vi "Load Tiff image from data.vi"(8 "Litt/BigEnd":bool, 9 "DirEntries":T1[](array[typedef]), 11 "Image Data in":u8[](array[numeric])) -> (1 "N_Bits":u64, 2 "Gray16/32":sgl[][](array[numeric]))   [LabVIEW 2013, in "Tiff reader.lvlib"]
doc: "This .vi loads a Tiff image from file."
uses:
  Tiff reader.lvlib
  IFD Entry.ctl
  FieldTypes.ctl
panel:
  in  "Tab Control":T3(tab)
  out "Gray8":u8[][](array[numeric])
  out "Grayscale":picture
  out "Gray8 LUT":u8[][](array[numeric])
  out "GrayWithLUT":picture
  out "RGB8":u32[][](array[numeric])
  out "B16/32":sgl[][](array[numeric])
  out "G16/32":sgl[][](array[numeric])
  out "R16/32":sgl[][](array[numeric])
  out "N_RGB_Bits":u64
  out "RGB":picture
  in  "error in (no error)":errorcluster
  out "error out":errorcluster
  out "PhotoM":T4(ring)=enum."BlackIsZero"
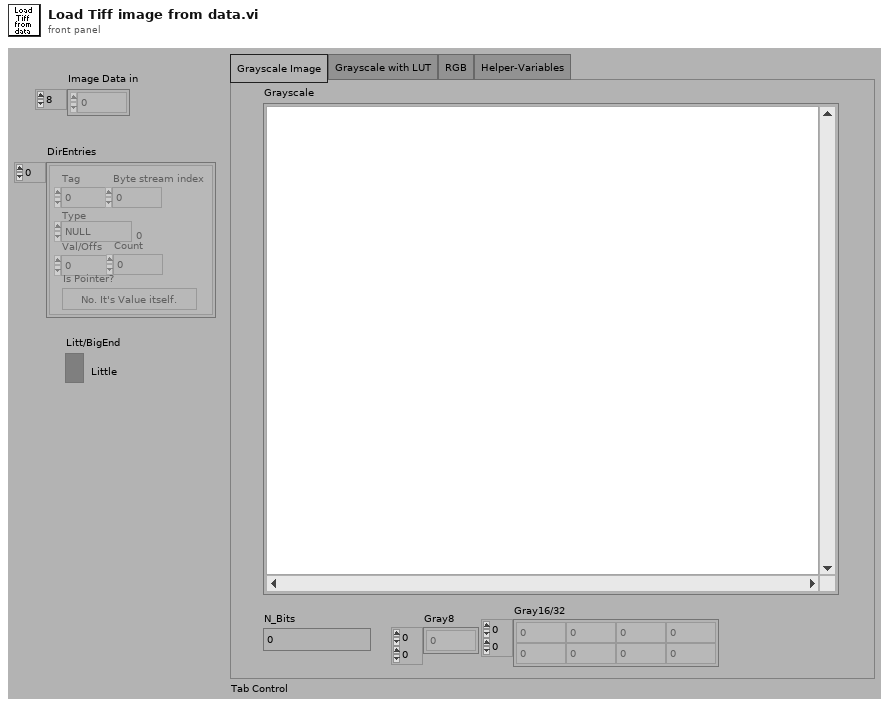
[diagram p1: front panel]
types:
  T1 = typedef "Tiff reader.lvlib/IFD Entry.ctl" = cluster{"Tag":u16, "Type":T2, "Count":u32, "Val/Offs":u32, "Is Pointer?":bool, "Byte stream index":i32}
  T2 = typedef "Tiff reader.lvlib/FieldTypes.ctl" = enum16{"NULL", "U8", "ASCII7", "U16", "U32", "RATIONAL", "SByte(I8)", "Undef(8Bit)", "I16", "I32", "SRat(4B:4B)", "SGL(4Byte)", "DBL(8Byte)"}
  T3 = enum32{"Grayscale Image", "Grayscale with LUT", "RGB", "Helper-Variables"}
  T4 = enum16{"WhiteIsZero", "BlackIsZero", "RGB", "RGBPalette", "TranspMask", "CMYK", "YCbCr", "Null", "CIELab"}
  T5 = typedef "imagedata.ctl" = cluster{"image type":i32, "image depth":i32, "image":u8[], "mask":u8[], "colors":u32[], "Rectangle":cluster{"left":i16, "top":i16, "right":i16, "bottom":i16}}
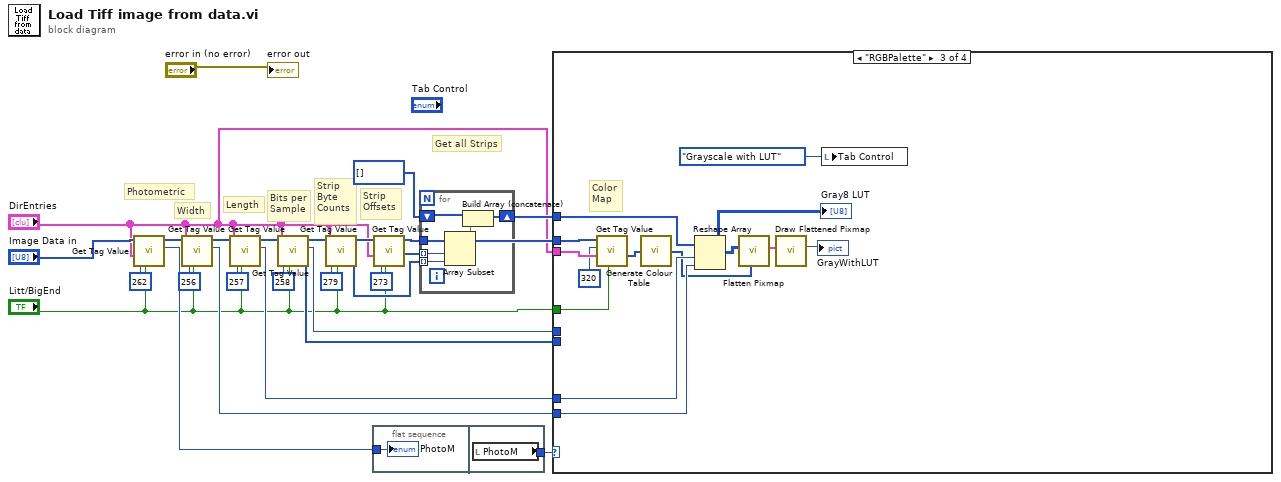
[diagram p0: block diagram]
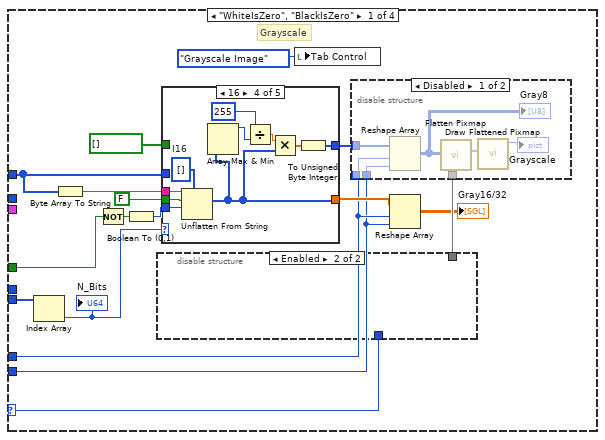
[diagram p2: hidden frame]
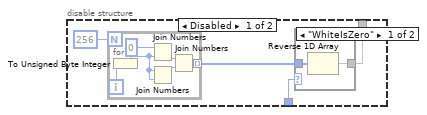
[diagram p3: hidden frame]
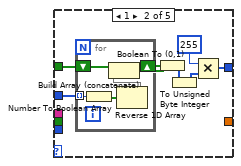
[diagram p7: hidden frame]
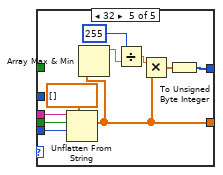
[diagram p9: hidden frame]
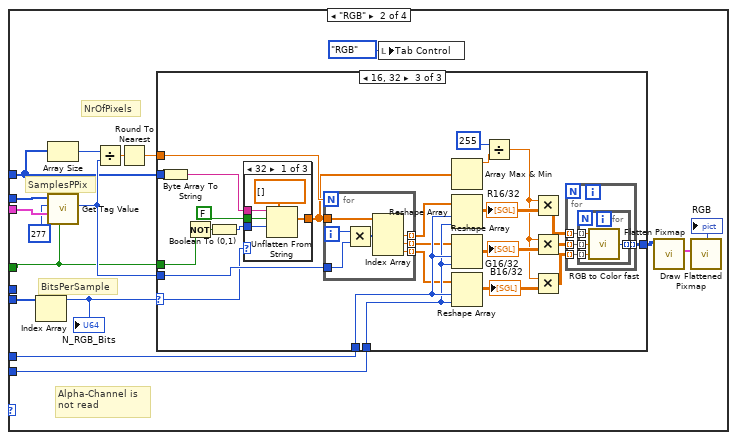
[diagram p10: hidden frame]
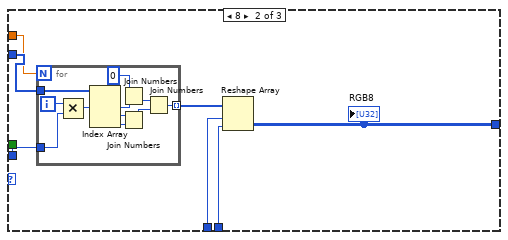
[diagram p12: hidden frame]
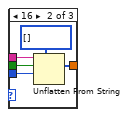
[diagram p13: hidden frame]
diagram:
  # "Get all Strips"
  # "Strip\nOffsets"
  # "Strip\nByte\nCounts"
  # "Bits per\nSample"
  # "Photometric"
  # "Length"
  # "Width"
  n1 = call "Get Tag Value.vi"("Litt/BigEnd"="Litt/BigEnd", "DirEntries"="DirEntries", "Tag Code"=u16 262, "Image Data in"="Image Data in") -> ("Single Value"=w11:u32, "Image Data out"=w21:u8[])  [unwired: 4 out]
  n2 = call "Get Tag Value.vi"("Litt/BigEnd"="Litt/BigEnd", "DirEntries"="DirEntries", "Tag Code"=u16 256, "Image Data in"=w21) -> ("Single Value"=w22:u32, "Image Data out"=w26:u8[])  [unwired: 4 out]
  n3 = call "Get Tag Value.vi"("Litt/BigEnd"="Litt/BigEnd", "DirEntries"="DirEntries", "Tag Code"=u16 257, "Image Data in"=w26) -> ("Single Value"=w23:u32, "Image Data out"=w18:u8[])  [unwired: 4 out]
  n4 = call "Get Tag Value.vi"("Litt/BigEnd"="Litt/BigEnd", "DirEntries"="DirEntries", "Tag Code"=u16 258, "Image Data in"=w18) -> ("Multiple Values"=w12:u64[], "Single Value"=w13:u32, "Image Data out"=w17:u8[])  [unwired: 3 out]
  n5 = call "Get Tag Value.vi"("Litt/BigEnd"="Litt/BigEnd", "DirEntries"="DirEntries", "Tag Code"=u16 279, "Image Data in"=w17) -> ("Multiple Values"=w7:u64[], "Image Data out"=w16:u8[])  [unwired: 4 out]
  n6 = flat-sequence {
    tunnel: w11 -> [w27]
    tunnel: [w28] -> w10
    frame #0 {
      "PhotoM" <- w27
    }
    frame #1 {
      n7 = local read "PhotoM"() -> (w28:T4)
    }
  }
  n8 = call "Get Tag Value.vi"("Litt/BigEnd"="Litt/BigEnd", "DirEntries"="DirEntries", "Tag Code"=u16 273, "Image Data in"=w16) -> ("Multiple Values"=w8:u64[], "Image Data out"=w9:u8[])  [unwired: 4 out]
  n9 = for {
    tunnel: w9 -> [w34]
    tunnel: w8 -> [w33] mode=indexing
    tunnel: w7 -> [w32] mode=indexing
    shift-right: [w31] -> w5
    shift-left: u8[] [] -> [w29]
    n10 = Array Subset(array=w34, index=w33, length=w32) -> (w30:u8[])
    n11 = Build Array (concatenate)(w29, w30) -> (w31:u8[])
  }
  n12 = case shown="\"RGBPalette\"" w10 {
    selector: w10 -> [w42 _ _ _]
    tunnel: w23 -> [w41 w121 w197 _]
    tunnel: w9 -> [_ w119 w199 _]
    tunnel: w22 -> [w40 w120 w196 _]
    tunnel: "DirEntries" -> [_ w118 w202 _]
    tunnel: w13 -> [_ _ _ _]
    tunnel: w12 -> [w47 w116 _ _]
    tunnel: w5 -> [w46 w107 w195 _]
    tunnel: "Litt/BigEnd" -> [w37 w105 w190 _]
    frame "WhiteIsZero", "BlackIsZero" {
      # "Grayscale"
      n13 = Index Array(array=w47) -> (element=w39:u64)  [unwired: 1 in]
      "N_Bits" <- w39
      n14 = Byte Array To String(unsigned byte array=w46) -> (string=w51:string)
      n15 = Not(x=w37) -> (.not. x?=w48:bool)
      n16 = Boolean To (0,1)(Boolean=w48) -> (0, 1=w49:i16)
      n17 = disable-structure shown="Enabled" {
        disable-tunnel: [w53 _] -> w43
        disable-tunnel: w42 -> [w52 _]
        frame Disabled {
          n18 = for {
            N: 256 -> [_]
            tunnel: [w59] -> w54 mode=indexing
            i -> [w64]
            n19 = To Unsigned Byte Integer(number=w64) -> (unsigned 8bit integer=w62:u8)
            n20 = Join Numbers(hi=u8 0, lo=w62) -> ((hi.lo)=w60:u16)
            n21 = Join Numbers(hi=w62, lo=w62) -> ((hi.lo)=w61:u16)
            n22 = Join Numbers(hi=w60, lo=w61) -> ((hi.lo)=w59:u32)
          }
          n23 = case shown="\"WhiteIsZero\"" w52 {
            tunnel: w54 -> [w57 w58]
            tunnel: [w56 w58] -> w53
            frame "WhiteIsZero" {
              n24 = Reverse 1D Array(array=w57) -> (reversed array=w56:u32[])
            }
            frame "BlackIsZero", Default {
            }
          }
        }
        frame Enabled {
        }
      }
      n25 = case shown="16" w39 {
        tunnel: w51 -> [_ _ _ w94 w103]
        tunnel: [_ _ w84 w85 w96] -> w44
        tunnel: FALSE ("data includes array or string size? (T)") -> [_ _ _ w93 w102]
        tunnel: w49 -> [_ _ _ w92 w101]
        tunnel: w46 -> [_ w78 w84 _ _]
        tunnel: [_ w73 w84 w86 w97] -> w45
        tunnel: bool[] [] -> [_ w72 _ _ _]
        frame 0, 4, Default {
          # "not\nsupported"
        }
        frame 1 {
          n26 = for {
            tunnel: w78 -> [w83] mode=indexing
            shift-right: [w82] -> w77
            shift-left: w72 -> [w81]
            n27 = Number To Boolean Array(number=w83) -> (Boolean array=w80:bool[])
            n28 = Reverse 1D Array(array=w80) -> (reversed array=w79:bool[])
            n29 = Build Array (concatenate)(w81, w79) -> (w82:bool[])
          }
          n30 = Boolean To (0,1)(Boolean=w77) -> (0, 1=w76:i16[])
          n31 = To Unsigned Byte Integer(number=w76) -> (unsigned 8bit integer=w75:u8[])
          n32 = Multiply(x=u8 255, y=w75) -> (x*y=w73:u8[])
        }
        frame 8 {
        }
        frame 16 {
          w91 = i16[] []  # I16
          n33 = Unflatten From String(type=w91, binary string=w94, data includes array or string size? (T)=w93, byte order (0:big-endian, network order)=w92) -> (value=w85:i16[])  [unwired: 1 in, 2 out]
          n34 = Array Max & Min(array=w85) -> (max value=w90:i16)  [unwired: 3 out]
          n35 = Divide(x=255 ("Numeric"), y=w90) -> (x/y=w89:dbl)
          n36 = Multiply(x=w89, y=w85) -> (x*y=w87:dbl[])
          n37 = To Unsigned Byte Integer(number=w87) -> (unsigned 8bit integer=w86:u8[])
        }
        frame 32 {
          n38 = Unflatten From String(type=sgl[] [], binary string=w103, data includes array or string size? (T)=w102, byte order (0:big-endian, network order)=w101) -> (value=w96:sgl[])  [unwired: 1 in, 2 out]
          n39 = Array Max & Min(array=w96) -> (max value=w100:sgl)  [unwired: 3 out]
          n40 = Divide(x=255 ("Numeric"), y=w100) -> (x/y=w99:sgl)
          n41 = Multiply(x=w99, y=w96) -> (x*y=w98:sgl[])
          n42 = To Unsigned Byte Integer(number=w98) -> (unsigned 8bit integer=w97:u8[])
        }
      }
      n43 = local write "Tab Control"(T3."Grayscale Image" ("Tab Control")) -> ()
      n44 = disable-structure shown="Disabled" {
        disable-tunnel: w45 -> [w71 _]
        disable-tunnel: w43 -> [w69 _]
        disable-tunnel: w41 -> [w68 _]
        disable-tunnel: w40 -> [w67 _]
        frame Disabled {
          n45 = Reshape Array(w71, w68, w67) -> (w65:u8[][])
          "Gray8" <- w65
          n46 = call <vilib>:"Flatten Pixmap.vi"("colors"=w69, "8-bit pixmap"=w65) -> ("image data"=w70:T5)  [unwired: 4 in, 5 out]
          n47 = call <vilib>:"Draw Flattened Pixmap.vi"("image data"=w70) -> ("new picture"=→"Grayscale":picture)  [unwired: 1 in, 7 out]
        }
        frame Enabled {
        }
      }
      n48 = Reshape Array(w44, w41, w40) -> (→"Gray16/32":sgl[][])
    }
    frame "RGB" {
      # "BitsPerSample"
      # "NrOfPixels"
      # "Alpha-Channel is\nnot read"
      # "SamplesPPix"
      n49 = Index Array(array=w116) -> (element=w111:u64)  [unwired: 1 in]
      "N_RGB_Bits" <- w111
      n50 = Array Size(array=w107) -> (size(s)=w106:i32)
      n51 = call "Get Tag Value.vi"("Litt/BigEnd"=w105, "DirEntries"=w118, "Tag Code"=u16 277, "Image Data in"=w119) -> ("Single Value"=w113:u32)  [unwired: 5 out]
      n52 = Divide(x=w106, y=w113) -> (x/y=w115:dbl)
      n53 = Round To Nearest(number=w115) -> (nearest integer value=w114:dbl)
      n54 = case shown="16, 32" w111 {
        selector: w111 -> [_ _ w156]
        tunnel: w121 -> [_ w127 w164]
        tunnel: w120 -> [_ w126 w163]
        tunnel: w113 -> [_ w125 w160]
        tunnel: w107 -> [_ w124 w155]
        tunnel: w114 -> [_ w123 w161]
        tunnel: [_ w122 w141] -> w108
        tunnel: w105 -> [_ _ w140]
        frame 0, Default {
        }
        frame 8 {
          n55 = for {
            N: w123 -> [_]
            tunnel: w124 -> [w139]
            tunnel: [w132] -> w128 mode=indexing
            tunnel: w125 -> [w129]
            i -> [w130]
            n56 = Multiply(x=w130, y=w129) -> (x*y=w131:u32)
            n57 = Index Array(array=w139, index #1=w131) -> (element #1=w138:u8, element #2=w137:u8, element #3=w136:u8)  [unwired: 2 in]
            n58 = Join Numbers(hi=u8 0, lo=w138) -> ((hi.lo)=w133:u16)
            n59 = Join Numbers(hi=w137, lo=w136) -> ((hi.lo)=w134:u16)
            n60 = Join Numbers(hi=w133, lo=w134) -> ((hi.lo)=w132:u32)
          }
          n61 = Reshape Array(w128, w127, w126) -> (w122:u32[][])
          "RGB8" <- w122
        }
        frame 16, 32 {
          n62 = Byte Array To String(unsigned byte array=w155) -> (string=w162:string)
          n63 = Not(x=w140) -> (.not. x?=w157:bool)
          n64 = Boolean To (0,1)(Boolean=w157) -> (0, 1=w158:i16)
          n65 = case shown="32" w156 {
            tunnel: w162 -> [w177 w182 _]
            tunnel: [w173 w181 _] -> w151
            tunnel: FALSE ("data includes array or string size? (T)") -> [w176 w180 _]
            tunnel: w158 -> [w175 w179 _]
            frame 32 {
              n66 = Unflatten From String(type=sgl[] [], binary string=w177, data includes array or string size? (T)=w176, byte order (0:big-endian, network order)=w175) -> (value=w173:sgl[])  [unwired: 1 in, 2 out]
            }
            frame 16 {
              n67 = Unflatten From String(type=u16[] [], binary string=w182, data includes array or string size? (T)=w180, byte order (0:big-endian, network order)=w179) -> (value=w181:u16[])  [unwired: 1 in, 2 out]
            }
            frame 0, Default {
            }
          }
          n68 = for {
            N: w161 -> [_]
            tunnel: w151 -> [w189]
            tunnel: [w188] -> w150 mode=indexing
            tunnel: [w187] -> w154 mode=indexing
            tunnel: [w186] -> w153 mode=indexing
            tunnel: w160 -> [w183]
            i -> [w184]
            n69 = Multiply(x=w184, y=w183) -> (x*y=w185:u32)
            n70 = Index Array(array=w189, index #1=w185) -> (element #1=w188:sgl, element #2=w187:sgl, element #3=w186:sgl)  [unwired: 2 in]
          }
          n71 = Array Max & Min(array=w151) -> (max value=w149:sgl)  [unwired: 3 out]
          n72 = Reshape Array(w150, w164, w163) -> (w148:sgl[][])
          "R16/32" <- w148
          n73 = Reshape Array(w154, w164, w163) -> (w147:sgl[][])
          "G16/32" <- w147
          n74 = Reshape Array(w153, w164, w163) -> (w146:sgl[][])
          "B16/32" <- w146
          n75 = Divide(x=255, y=w149) -> (x/y=w145:sgl)
          n76 = Multiply(x=w145, y=w148) -> (x*y=w144:sgl[][])
          n77 = Multiply(x=w145, y=w147) -> (x*y=w143:sgl[][])
          n78 = Multiply(x=w145, y=w146) -> (x*y=w142:sgl[][])
          n79 = for {
            tunnel: w144 -> [w168] mode=indexing
            tunnel: w143 -> [w167] mode=indexing
            tunnel: w142 -> [w166] mode=indexing
            tunnel: [w165] -> w141 mode=indexing
            n80 = for {
              tunnel: w168 -> [w172] mode=indexing
              tunnel: w167 -> [w171] mode=indexing
              tunnel: w166 -> [w170] mode=indexing
              tunnel: [w169] -> w165 mode=indexing
              n81 = call "RGB to Color fast.vi"("B"=w170, "G"=w171, "R"=w172) -> ("Color"=w169:u32)
            }
          }
        }
      }
      n82 = local write "Tab Control"(T3."RGB" ("Tab Control")) -> ()
      n83 = call <vilib>:"Flatten Pixmap.vi"("24-bit pixmap"=w108) -> ("image data"=w109:T5)  [unwired: 5 in, 5 out]
      n84 = call <vilib>:"Draw Flattened Pixmap.vi"("image data"=w109) -> ("new picture"=→"RGB":picture)  [unwired: 1 in, 7 out]
    }
    frame "RGBPalette" {
      # "Color\nMap"
      n85 = call "Get Tag Value.vi"("Litt/BigEnd"=w190, "DirEntries"=w202, "Tag Code"=u16 320, "Image Data in"=w199) -> ("Multiple Values"=w201:u64[])  [unwired: 5 out]
      n86 = call "Generate Colour Table.vi"("Code 320 Values"=w201) -> ("Colour Table"=w194:u32[])
      n87 = Reshape Array(w195, w197, w196) -> (w191:u8[][])
      "Gray8 LUT" <- w191
      n88 = call <vilib>:"Flatten Pixmap.vi"("colors"=w194, "8-bit pixmap"=w191) -> ("image data"=w198:T5)  [unwired: 4 in, 5 out]
      n89 = call <vilib>:"Draw Flattened Pixmap.vi"("image data"=w198) -> ("new picture"=→"GrayWithLUT":picture)  [unwired: 1 in, 7 out]
      n90 = local write "Tab Control"(T3."Grayscale with LUT" ("Tab Control")) -> ()
    }
    frame "TranspMask".."CIELab" {
      # "unsupported"
    }
  }
  "error out" <- "error in (no error)"
